vi "MotionControl.vi"(5 "Frequency (Hz) 3":u32=650 format="%.2f", 7 "Motion Type":enum16{"Linear", "Rotational"}(ring), 8 "Error In":errorcluster, 9 "Distance":dbl, 10 "Direction":bool, 11 "AirSAS Controls":T1={"Receive Duration"=0.0, "I/O"={"DAQmx Device"="Dev1", "AO Range"=0.0, "AI Range"=0.0, "DAQ Group Delay"=0.0, "Fs"=0.0}, "Hardware"={"Centerpos"=[], "TXpos"=[], "RX1pos"=[], "RX2pos"=[], "Angle"=0.0, "Height"=0.0}, "Waveform"={"LFM Parameters"={"Duration"=1.0, "Fstart (Hz)"=1000.0, "Fstop (Hz)"=10000.0, "Out. Amplitude (Vpk)"=1.0, "Window %"=10.0}, "Transmit Waveform"={"t0"=timestamp(0 s since 1904-01-01), "dt"=1.0, "Y"=[]}}, "LINX Resource"={"IO"=enum."Remote", "Interface"=enum."Serial", "LINX Device Config"={"Interface"=enum."Serial", "COM Port"="COM13", "TCP Configuration"={"IP Address"="", "Port"=0}, "Device Family"=1, "Device ID"=1, "Device Name"="myRIO-1900", "TCP Ref"=refnum, "Channels"={"DI"=[0, 1, 2, 3, 4, 5, 6, 7, 8, 9, 10, 11, 12, 13, 14, 15, 16, 17, 18, 19, 20, 21, 22, 23, 24, 25, 26, 27, 28, 29, 30, 31, 32, 33, 34, 35, 36, 37, 38, 39, 40, 41, 42, 43, 44, 45, 46], "DO"=[0, 1, 2, 3, 4, 5, 6, 7, 8, 9, 10, 11, 12, 13, 14, 15, 16, 17, 18, 19, 20, 21, 22, 23, 24, 25, 26, 27, 28, 29, 30, 31, 32, 33, 34, 35, 36, 37, 38, 39, 40, 41, 42, 43, 44, 45, 46], "AI"=[0, 1, 2, 3, 4, 5, 6, 7, 8, 9, 10, 11], "AO"=[], "PWM"=[3, 5, 6, 9, 10], "QE"=[], "UART"=[0, 1], "I2C 2"=[0], "SPI"=[0], "CAN"=[], "Servo"=[], "AI Ref (V)"=0.0, "AI Resolution (Bits)"=0, "AO Ref (V)"=0.0, "AO Resolution (Bits)"=0}}}, "Port"=3000.0} {"Waveform"."LFM Parameters"."Window %" format="%.2g"; "Waveform"."LFM Parameters"."Out. Amplitude (Vpk)" format="%0.2f"; "Waveform"."LFM Parameters"."Fstop (Hz)" format="%^.3e"; "Waveform"."LFM Parameters"."Fstart (Hz)" format="%^.3e"; "Waveform"."LFM Parameters"."Duration" format="%.3f"}) -> (0 "Error Out":errorcluster, 3 "output cluster":T1={"Receive Duration"=0.0, "I/O"={"DAQmx Device"="Dev1", "AO Range"=0.0, "AI Range"=0.0, "DAQ Group Delay"=0.0, "Fs"=0.0}, "Hardware"={"Centerpos"=[0.0, 0.0, 0.0], "TXpos"=[0.0, 0.0, 0.0], "RX1pos"=[0.0, 0.0, 0.0], "RX2pos"=[0.0, 0.0, 0.0], "Angle"=0.0, "Height"=0.0}, "Waveform"={"LFM Parameters"={"Duration"=1.0, "Fstart (Hz)"=1000.0, "Fstop (Hz)"=10000.0, "Out. Amplitude (Vpk)"=1.0, "Window %"=10.0}, "Transmit Waveform"={"t0"=timestamp(0 s since 1904-01-01), "dt"=1.0, "Y"=[]}}, "LINX Resource"={"IO"=enum."Remote", "Interface"=enum."Serial", "LINX Device Config"={"Interface"=enum."Serial", "COM Port"="COM13", "TCP Configuration"={"IP Address"="", "Port"=0}, "Device Family"=1, "Device ID"=1, "Device Name"="myRIO-1900", "TCP Ref"=refnum, "Channels"={"DI"=[0, 1, 2, 3, 4, 5, 6, 7, 8, 9, 10, 11, 12, 13, 14, 15, 16, 17, 18, 19, 20, 21, 22, 23, 24, 25, 26, 27, 28, 29, 30, 31, 32, 33, 34, 35, 36, 37, 38, 39, 40, 41, 42, 43, 44, 45, 46], "DO"=[0, 1, 2, 3, 4, 5, 6, 7, 8, 9, 10, 11, 12, 13, 14, 15, 16, 17, 18, 19, 20, 21, 22, 23, 24, 25, 26, 27, 28, 29, 30, 31, 32, 33, 34, 35, 36, 37, 38, 39, 40, 41, 42, 43, 44, 45, 46], "AI"=[0, 1, 2, 3, 4, 5, 6, 7, 8, 9, 10, 11], "AO"=[], "PWM"=[3, 5, 6, 9, 10], "QE"=[], "UART"=[0, 1], "I2C 2"=[0], "SPI"=[0], "CAN"=[], "Servo"=[], "AI Ref (V)"=0.0, "AI Resolution (Bits)"=0, "AO Ref (V)"=0.0, "AO Resolution (Bits)"=0}}}, "Port"=3000.0} {"Waveform"."LFM Parameters"."Window %" format="%.2g"; "Waveform"."LFM Parameters"."Out. Amplitude (Vpk)" format="%0.2f"; "Waveform"."LFM Parameters"."Fstop (Hz)" format="%^.3e"; "Waveform"."LFM Parameters"."Fstart (Hz)" format="%^.3e"; "Waveform"."LFM Parameters"."Duration" format="%.3f"})   [LabVIEW 2021]
uses:
  controls/Air SAS Controls.ctl
  <vilib>/MakerHub/LINX/Private/Type Defs/LINX Ref.ctl
  <vilib>/MakerHub/LINX/Private/Type Defs/Platform.ctl
  <vilib>/MakerHub/LINX/Private/Type Defs/Interface.ctl
  <vilib>/MakerHub/LINX/Private/Device/Type Defs/LINX Device Config.ctl
  <vilib>/MakerHub/LINX/Private/Device/Type Defs/TCP Config.ctl
  <vilib>/MakerHub/LINX/Private/Device/Type Defs/Channels.ctl
  <vilib>/Utility/error.llb/DialogType.ctl
  <vilib>/MakerHub/LINX/Public/Peripherals/Digital/Digital Write 1 Chan.vi
  <vilib>/MakerHub/LINX/Public/Peripherals/Digital/Digital Write N Chans.vi
  <vilib>/MakerHub/LINX/Private/Local IO/LinxDigitalWrite.vi
  <vilib>/MakerHub/LINX/Public/Utilities/Check Channel.vi
  <vilib>/MakerHub/LINX/Private/Utilties/Generate Error.vi
  <vilib>/MakerHub/LINX/LMH-LINX.lvlib
  <vilib>/MakerHub/LINX/Private/Device/Device.lvlib
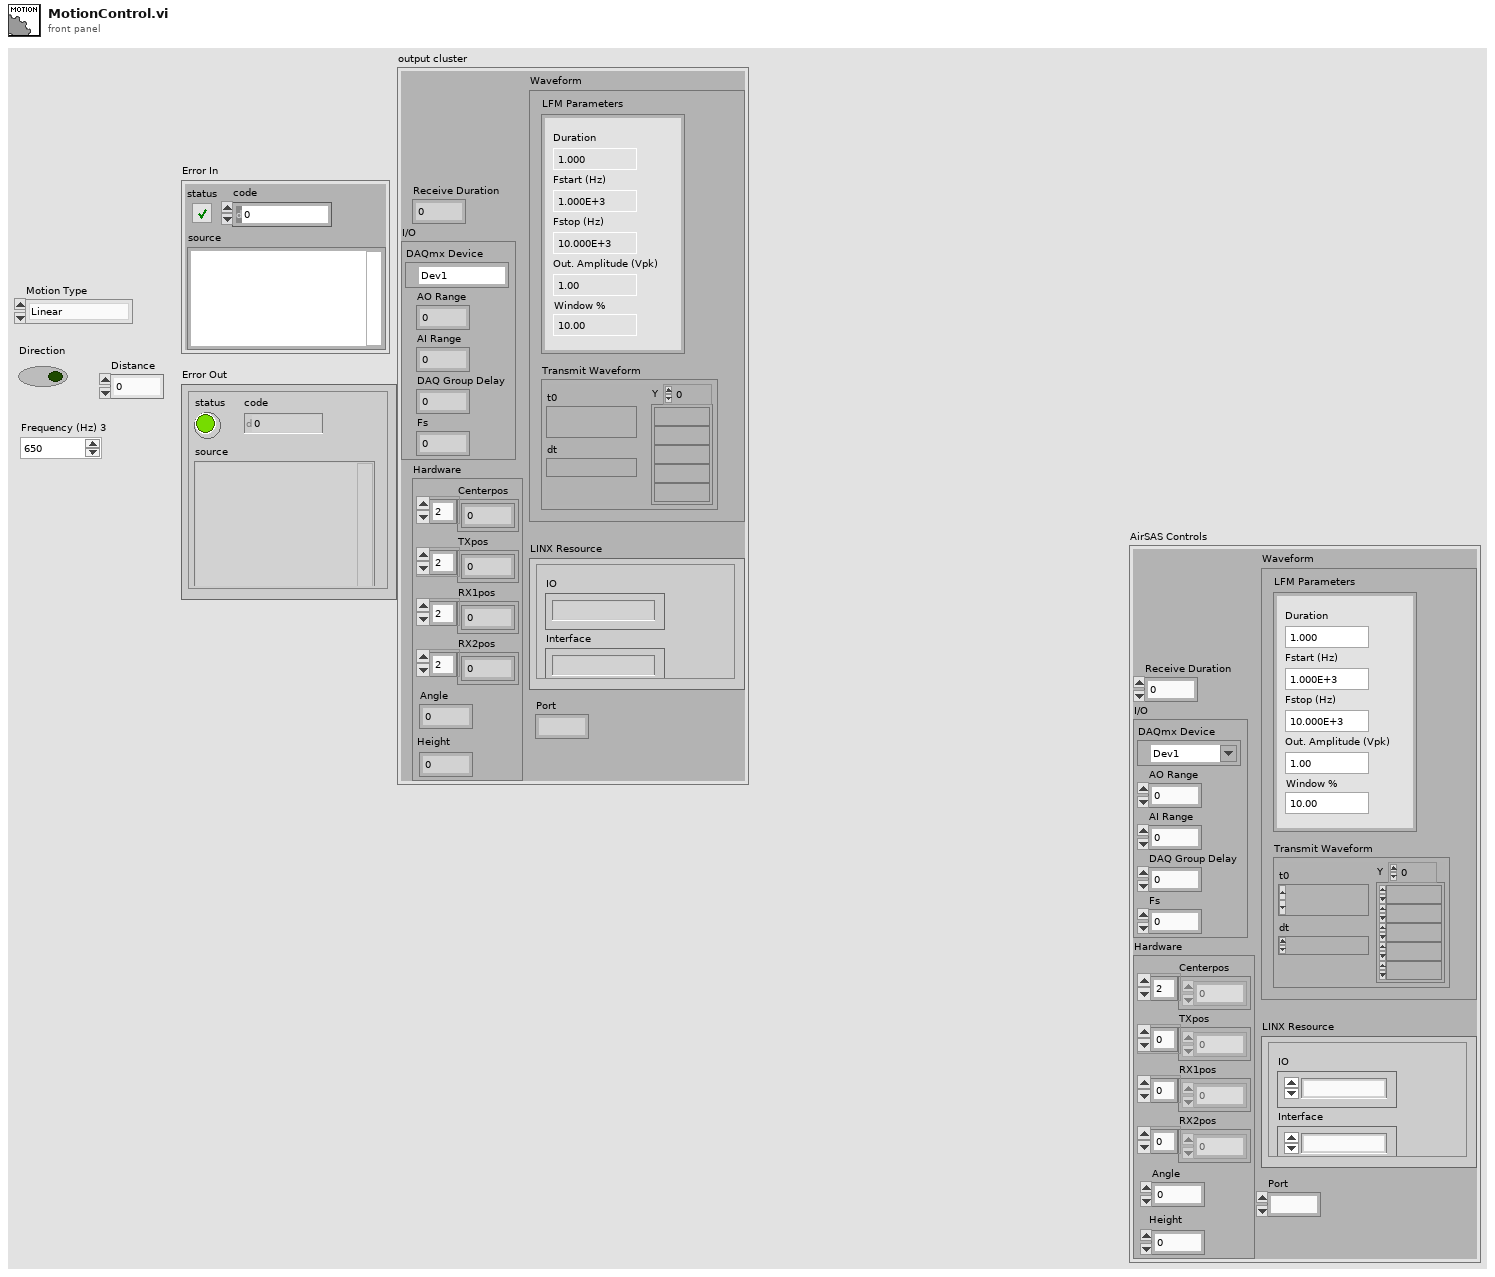
[diagram p1: front panel]
types:
  T1 = typedef "Air SAS Controls.ctl" = cluster{"Receive Duration":dbl, "I/O":cluster{"DAQmx Device":tag, "AO Range":dbl, "AI Range":dbl, "DAQ Group Delay":dbl, "Fs":dbl}, "Hardware":cluster{"Centerpos":dbl[], "TXpos":dbl[], "RX1pos":dbl[], "RX2pos":dbl[], "Angle":dbl, "Height":dbl}, "Waveform":cluster{"LFM Parameters":cluster{"Duration":dbl, "Fstart (Hz)":dbl, "Fstop (Hz)":dbl, "Out. Amplitude (Vpk)":dbl, "Window %":dbl}, "Transmit Waveform":waveform(dbl)}, "LINX Resource":T2, "Port":dbl}
  T2 = typedef "LMH-LINX.lvlib/LINX Ref.ctl" = cluster{"IO":T3, "Interface":T4, "LINX Device Config":T5}
  T3 = typedef "LMH-LINX.lvlib/Platform.ctl" = enum16{"Remote", "Local"}
  T4 = typedef "LMH-LINX.lvlib/Interface.ctl" = enum16{"Serial", "TCP"}
  T5 = typedef "LMH-LINX.lvlib/Device.lvlib/LINX Device Config.ctl" = cluster{"Interface":T4, "COM Port":refnum<visa-resource-name>, "TCP Configuration":T6, "Device Family":u8, "Device ID":u8, "Device Name":string, "TCP Ref":refnum<k5>, "Channels":T7}
  T6 = typedef "LMH-LINX.lvlib/Device.lvlib/TCP Config.ctl" = cluster{"IP Address":string, "Port":u16}
  T7 = typedef "LMH-LINX.lvlib/Channels.ctl" = cluster{"DI":u8[], "DO":u8[], "AI":u8[], "AO":u8[], "PWM":u8[], "QE":u8[], "UART":u8[], "I2C 2":u8[], "SPI":u8[], "CAN":u8[], "Servo":u8[], "AI Ref (V)":dbl, "AI Resolution (Bits)":u8, "AO Ref (V)":dbl, "AO Resolution (Bits)":u8}
  T8 = typedef "DialogType.ctl" = u16
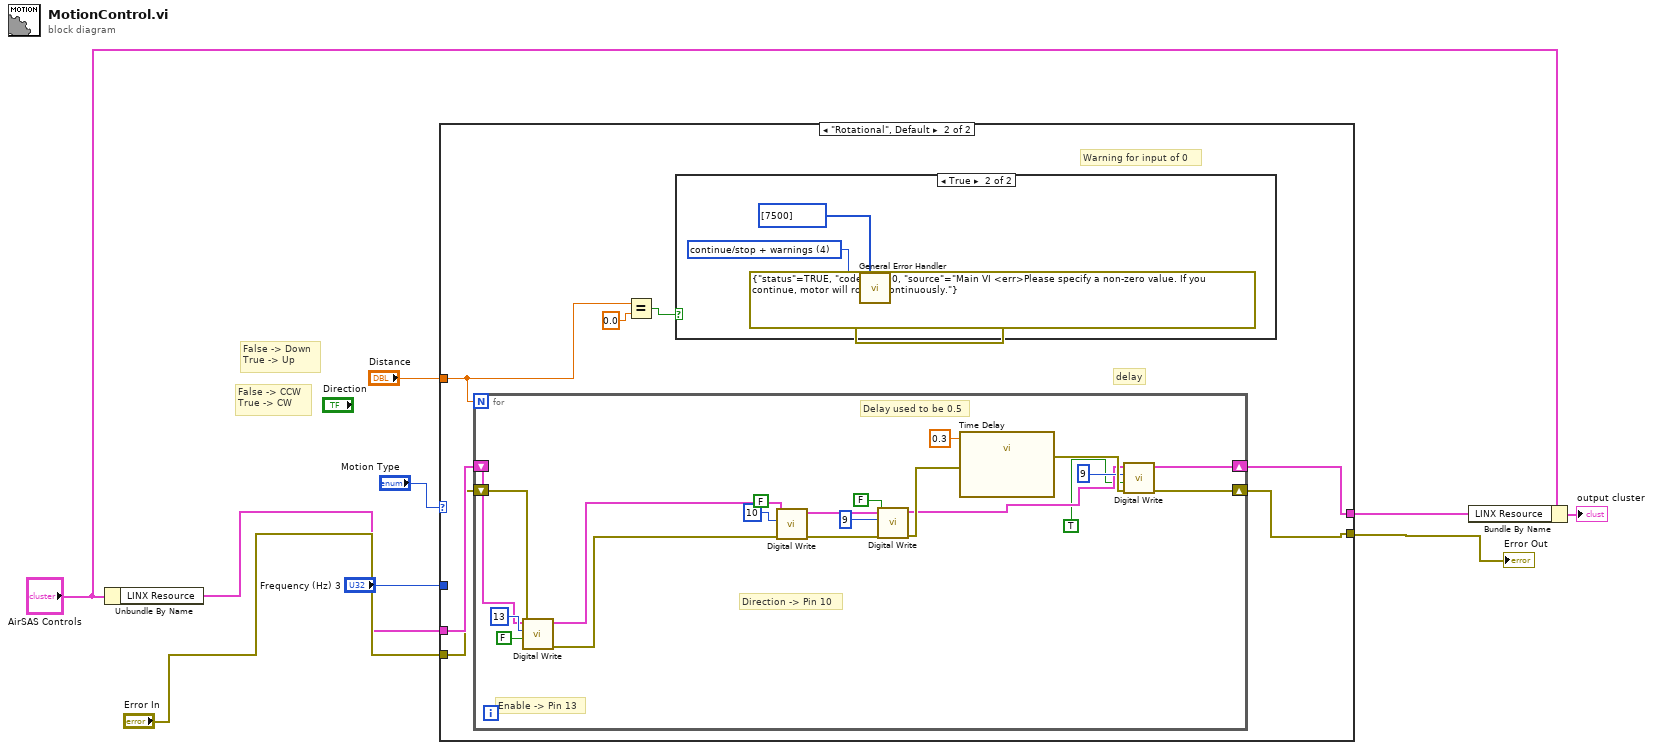
[diagram p0: block diagram]
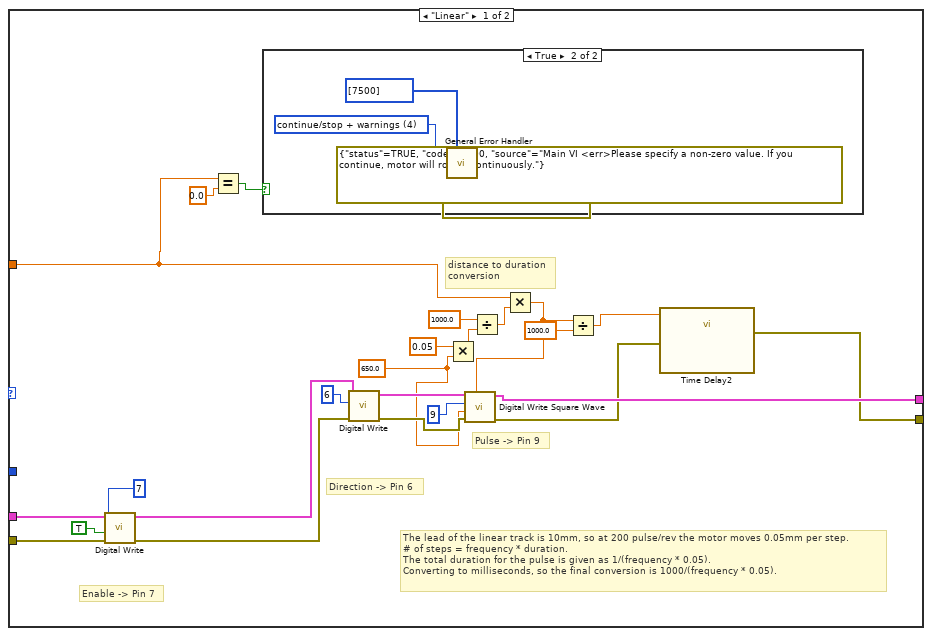
[diagram p2: hidden frame]
diagram:
  # "False -> CCW\nTrue -> CW"
  # "False -> Down\nTrue -> Up"
  n1 = Unbundle By Name("AirSAS Controls") -> ("LINX Resource"=w8:T2)
  n2 = case shown="\"Rotational\", Default" "Motion Type" {
    tunnel: w8 -> [w22 w43]
    tunnel: "Distance" -> [w16 w37]
    tunnel: [w26 w38] -> w5
    tunnel: "Error In" -> [w21 w42]
    tunnel: [w11 w39] -> w7
    tunnel: "Frequency (Hz) 3" -> [_ _]
    frame "Linear" {
      w10 = 650.0 ("y")
      # "The lead of the linear track is 10mm, so at 200 pulse/rev the motor moves 0.05mm per step. \n# of steps = frequency * duration.\nThe total duration for the pulse is given as 1/(frequency * 0.05).\nConverting to milliseconds, so the final conversion is 1000/(frequency * 0.05)."
      # "distance to duration\nconversion"
      # "Pulse -> Pin 9"
      # "Enable -> Pin 7"
      # "Direction -> Pin 6"
      n3 = call-poly <vilib>:"Digital Write.vi"("Error In"=w21, "Output Value"=TRUE, "DO Channel"=u8 7, "LINX Resource"=w22) -> ("Error Out"=w19:errorcluster, "LINX Resource"=w20:T2)  [unwired: 6 in]
      n4 = Equal?(x=w16, y=0.0) -> (x = y?=w18:bool)
      n5 = case shown="True" w18 {
        frame False {
        }
        frame True {
          w35 = T8 4 items=["no dialog", "OK message", "continue or stop message", "OK message + warnings", "continue/stop + warnings"] ("type of dialog (OK msg:1)")
          n6 = call <vilib>:"General Error Handler.vi"("[user-defined codes]"=i32[] [7500], "type of dialog (OK msg:1)"=w35, "error in (no error)"=errorcluster {"status"=TRUE, "code"=7500, "source"="Main VI <err>Please specify a non-zero value. If you continue, motor will rotate continuously."}) -> ()  [unwired: 8 in, 5 out]
        }
      }
      n7 = call-poly <vilib>:"Digital Write.vi"("Error In"=w19, "DO Channel"=u8 6 ("DIR channel"), "LINX Resource"=w20) -> ("Error Out"=w25:errorcluster, "LINX Resource"=w32:T2)  [unwired: 7 in]
      n8 = Multiply(x=0.05 ("y"), y=w10) -> (x*y=w29:dbl)
      n9 = Divide(x=1000.0, y=w29) -> (x/y=w27:dbl)
      n10 = Multiply(x=w16, y=w27) -> (x*y=w15:dbl)
      n11 = call <vilib>:"Digital Write Square Wave.vi"("Duration (ms)"=w15, "Error In"=w25, "Frequency (Hz)"=w10, "Channel"=u8 9 ("Digital Output Channel"), "LINX Resource"=w32) -> ("Error Out"=w12:errorcluster, "LINX Resource"=w26:T2)  [unwired: 5 in]
      n12 = Divide(x=w15, y=1000.0) -> (x/y=w13:dbl)
      n13 = call "Time Delay2"("error in (no error)"=w12, "Delay Time (s)"=w13) -> ("error out"=w11:errorcluster)  [unwired: 9 in]
    }
    frame "Rotational", Default {
      # "delay"
      # "Warning for input of 0"
      n14 = for {
        N: w37 -> [_]
        shift-right: [w46] -> w38
        shift-left: w43 -> [w58]
        shift-right: [w49] -> w39
        shift-left: w42 -> [w57]
        # "Delay used to be 0.5"
        # "Direction -> Pin 10"
        # "Enable -> Pin 13"
        n15 = call-poly <vilib>:"Digital Write.vi"("Error In"=w57, "Output Value"=FALSE, "DO Channel"=u8 13, "LINX Resource"=w58) -> ("Error Out"=w63:errorcluster, "LINX Resource"=w62:T2)  [unwired: 6 in]
        n16 = call-poly <vilib>:"Digital Write.vi"("Error In"=w63, "Output Value"=FALSE, "DO Channel"=u8 10 ("DIR channel"), "LINX Resource"=w62) -> ("Error Out"=w55:errorcluster, "LINX Resource"=w56:T2)  [unwired: 6 in]
        n17 = call-poly <vilib>:"Digital Write.vi"("Error In"=w55, "Output Value"=FALSE, "DO Channel"=u8 9, "LINX Resource"=w56) -> ("Error Out"=w52:errorcluster, "LINX Resource"=w47:T2)  [unwired: 6 in]
        n18 = call "Time Delay"("error in (no error)"=w52, "Delay Time (s)"=0.3) -> ("error out"=w50:errorcluster)  [unwired: 9 in]
        n19 = call-poly <vilib>:"Digital Write.vi"("Error In"=w50, "Output Value"=TRUE, "DO Channel"=u8 9, "LINX Resource"=w47) -> ("Error Out"=w49:errorcluster, "LINX Resource"=w46:T2)  [unwired: 6 in]
      }
      n20 = Equal?(x=w37, y=0.0) -> (x = y?=w40:bool)
      n21 = case shown="True" w40 {
        frame False {
        }
        frame True {
          w65 = T8 4 items=["no dialog", "OK message", "continue or stop message", "OK message + warnings", "continue/stop + warnings"] ("type of dialog (OK msg:1)")
          n22 = call <vilib>:"General Error Handler.vi"("[user-defined codes]"=i32[] [7500], "type of dialog (OK msg:1)"=w65, "error in (no error)"=errorcluster {"status"=TRUE, "code"=7500, "source"="Main VI <err>Please specify a non-zero value. If you continue, motor will rotate continuously."}) -> ()  [unwired: 8 in, 5 out]
        }
      }
    }
  }
  "Error Out" <- w7
  n23 = Bundle By Name(cluster="AirSAS Controls", "LINX Resource"=w5) -> (→"output cluster":T1)
